vi "NewtonsPSM_Conf_Generator.vi"(6 "Amplitude (2)":dbl=2.0 min=0.0 max=10.0 step=1e-05, 7 "Frequency (1000)":dbl=1000.0 min=0.0 max=35000000.0 step=0.0001, 8 "error in":errorcluster, 9 "Waveform (Sinewave)":enum16{"Sinewave", "Square"}(ring), 10 "Offset (0)":dbl min=-10.0 max=10.0 step=0.0001, 11 "VISA.name":refnum<visa-resource-name>) -> (0 "error out":errorcluster, 3 "VISA.name out":refnum<visa-resource-name>)   [LabVIEW 2025, in "NewtonsPSM1735.lvlib"]
doc: "This VI set the Special mode of the PPA2530."
uses:
  NewtonsPSM1735.lvlib
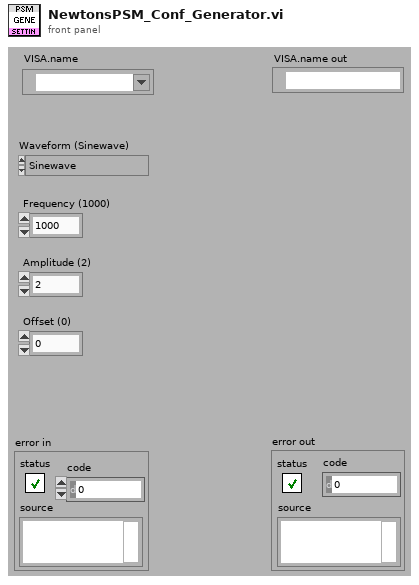
[diagram p1: front panel]
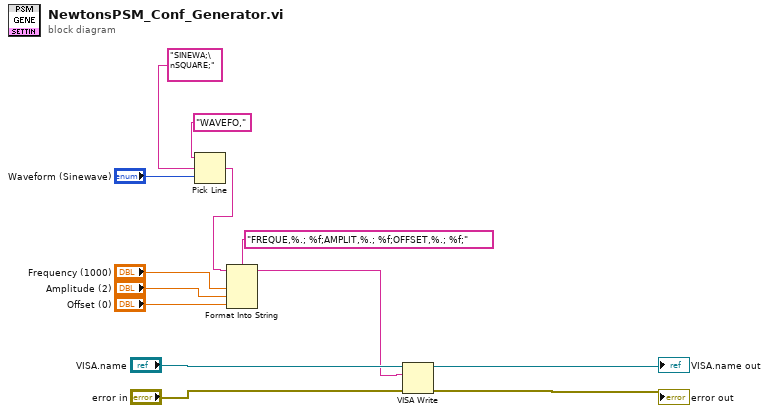
[diagram p0: block diagram]
diagram:
  n1 = Pick Line(string ("")="WAVEFO,", multi-line string="SINEWA;\nSQUARE;", line index="Waveform (Sinewave)") -> (output string=w2:string)
  n2 = Format Into String(format string="FREQUE,%.; %f;AMPLIT,%.; %f;OFFSET,%.; %f;" ("chaîne de format"), initial string=w2, "Frequency (1000)", "Amplitude (2)", "Offset (0)") -> (resulting string=w1:string)  [unwired: 1 in, 1 out]
  n3 = VISA Write(VISA resource name="VISA.name", write buffer=w1, error in (no error)="error in") -> (VISA resource name out=→"VISA.name out":refnum<visa-resource-name>, error out=→"error out":errorcluster)  [unwired: 1 out]
